vi "Engine-RPC-Host.vi"() -> ()   [LabVIEW 2016]
uses:
  Shared/Typedefs/Engine-RPC-Sync-Controls.ctl
  Shared/Typedefs/Engine-RPC-Sync-Indicators.ctl
  <vilib>/Powertrain Controls/Device Drivers/DCM/Rev0/FPGA/Digital Channel.ctl
  Shared/Typedefs/Engine-RPC-PWM-Controls.ctl
  Shared/Typedefs/Engine-RPC-PWM-Indicators.ctl
  <vilib>/addons/Software Calibration Management/XControls/SubHost.xctl
  Shared/Typedefs/UserParameter-Array.ctl
  Shared/Typedefs/UserParameter.ctl
  Shared/Typedefs/Engine-RPC-Modes.ctl
  Shared/Typedefs/Engine-Channel.ctl
  Shared/DSI-Shared.lvlib
  <vilib>/Powertrain Controls/Device Drivers/DCM/Rev0/FPGA/DCM - FPGA.lvlib
panel:
  in  "Mode":T1
  in  "_Hidden":enum32{"Page 1"}(tab)
  in  "_Refresh":bool
  out "PWM-A_Fault":bool
  out "PWM-B_Fault":bool
  out "Sync-A_Fault":bool
  out "Sync-B_Fault":bool
  out "PWM-A_DisHHChans":sgl[](array[numeric])
  out "PWM-B_DisHHChans":sgl[](array[numeric])
  out "Channels|Names":string[](array[string])
  in  "ENG|RPC|ClearFaults":bool
  out "ENG|RPC|Fault":bool caption="RailP"
  out "ENG|RPC|UserParamNames":string[](array[string])
  in  "ENG|RPC|UserParamValues":sgl[](array[numeric])
  out "ENG|RPC|UserResults":T2=[{"Name"="", "Value"=0.0}, {"Name"="", "Value"=0.0}, {"Name"="", "Value"=0.0}, {"Name"="", "Value"=0.0}, {"Name"="", "Value"=0.0}, {"Name"="", "Value"=0.0}, {"Name"="", "Value"=0.0}, {"Name"="", "Value"=0.0}, {"Name"="", "Value"=0.0}, {"Name"="", "Value"=0.0}, {"Name"="", "Value"=0.0}, {"Name"="", "Value"=0.0}, {"Name"="", "Value"=0.0}, {"Name"="", "Value"=0.0}, {"Name"="", "Value"=0.0}, {"Name"="", "Value"=0.0}, {"Name"="", "Value"=0.0}, {"Name"="", "Value"=0.0}, {"Name"="", "Value"=0.0}, {"Name"="", "Value"=0.0}, {"Name"="", "Value"=0.0}, {"Name"="", "Value"=0.0}, {"Name"="", "Value"=0.0}, {"Name"="", "Value"=0.0}, {"Name"="", "Value"=0.0}, {"Name"="", "Value"=0.0}, {"Name"="", "Value"=0.0}, {"Name"="", "Value"=0.0}, {"Name"="", "Value"=0.0}, {"Name"="", "Value"=0.0}, {"Name"="", "Value"=0.0}, {"Name"="", "Value"=0.0}, {"Name"="", "Value"=0.0}, {"Name"="", "Value"=0.0}, {"Name"="", "Value"=0.0}, {"Name"="", "Value"=0.0}, {"Name"="", "Value"=0.0}, {"Name"="", "Value"=0.0}, {"Name"="", "Value"=0.0}, {"Name"="", "Value"=0.0}, {"Name"="", "Value"=0.0}, {"Name"="", "Value"=0.0}, {"Name"="", "Value"=0.0}, {"Name"="", "Value"=0.0}, {"Name"="", "Value"=0.0}, {"Name"="", "Value"=0.0}, {"Name"="", "Value"=0.0}, {"Name"="", "Value"=0.0}, {"Name"="", "Value"=0.0}, {"Name"="", "Value"=0.0}, {"Name"="", "Value"=0.0}, {"Name"="", "Value"=0.0}, {"Name"="", "Value"=0.0}, {"Name"="", "Value"=0.0}, {"Name"="", "Value"=0.0}, {"Name"="", "Value"=0.0}, {"Name"="", "Value"=0.0}, {"Name"="", "Value"=0.0}, {"Name"="", "Value"=0.0}, {"Name"="", "Value"=0.0}, {"Name"="", "Value"=0.0}, {"Name"="", "Value"=0.0}, {"Name"="", "Value"=0.0}, {"Name"="", "Value"=0.0}, {"Name"="", "Value"=0.0}, {"Name"="", "Value"=0.0}, {"Name"="", "Value"=0.0}, {"Name"="", "Value"=0.0}, {"Name"="", "Value"=0.0}, {"Name"="", "Value"=0.0}, {"Name"="", "Value"=0.0}, {"Name"="", "Value"=0.0}, {"Name"="", "Value"=0.0}, {"Name"="", "Value"=0.0}, {"Name"="", "Value"=0.0}, {"Name"="", "Value"=0.0}, {"Name"="", "Value"=0.0}, {"Name"="", "Value"=0.0}, {"Name"="", "Value"=0.0}, {"Name"="", "Value"=0.0}, {"Name"="", "Value"=0.0}, {"Name"="", "Value"=0.0}, {"Name"="", "Value"=0.0}, {"Name"="", "Value"=0.0}, {"Name"="", "Value"=0.0}, {"Name"="", "Value"=0.0}, {"Name"="", "Value"=0.0}, {"Name"="", "Value"=0.0}, {"Name"="", "Value"=0.0}, {"Name"="", "Value"=0.0}, {"Name"="", "Value"=0.0}, {"Name"="", "Value"=0.0}, {"Name"="", "Value"=0.0}, {"Name"="", "Value"=0.0}, {"Name"="", "Value"=0.0}, {"Name"="", "Value"=0.0}, {"Name"="", "Value"=0.0}, {"Name"="", "Value"=0.0}, {"Name"="", "Value"=0.0}, {"Name"=" ", "Value"=0.0}]
  in  "Rail Pressure Plot":T4(xcontrol)={"Name"="Engine-RPC-Plot-Host (Engine-RPC-Plot-Host)", "Host VI"=path "Engine-RPC-Plot-Host.vi", "Pairing File"=path "Engine-RPC-Plot-Host.par", "Display Name"="Rail Pressure Plot"}
  in  "_RailP Summary Table":i32(listbox) caption="Summary"
  in  "_MainTab":T5(tab)
  in  "PWM-A_Controls":T6
  out "PWM-A_Indicators":T7={"IMV"={"Current_Calc"=0.0, "DutyCyc_PIDOut"=0.7671859, "DutyCyc_MaxCalc"=0.0, "DutyCyc_Des"=0.7671859}, "HPV"={"Current_Calc"=0.0, "DutyCyc_TblOut"=0.7671859, "DutyCyc_MaxCalc"=0.0, "DutyCyc_Des"=0.7671859}} {"HPV"."DutyCyc_Des" format="%#.3g"; "HPV"."DutyCyc_MaxCalc" max=50 format="%#.3g"; "HPV"."DutyCyc_TblOut" format="%#.3g"; "HPV"."Current_Calc" min=0 max=0.2 step=0.001 format="%#.3f"; "IMV"."DutyCyc_Des" format="%#.3g"; "IMV"."DutyCyc_MaxCalc" max=50 format="%#.3g"; "IMV"."DutyCyc_PIDOut" format="%#.3g"; "IMV"."Current_Calc" min=0 max=0.2 step=0.001 format="%#.3f"}
  in  "PWM-A_RailPStp":sgl caption="[bar]"
  out "_PWM-A_SetpointUnit":string
  out "_PWM-A_MaxUnit":string
  in  "PWM-A_MaxRailP":sgl caption="[bar]"
  in  "PWM-A_HPV_E":bool
  in  "PWM-A_IMV_E":bool
  in  "PWM-A_IMVPID_E":bool
  in  "_PWM-A_Tab":enum32{"Analog Inputs", "HH Outputs"}(tab)
  in  "PWM-A_RailPIndex":i32(ring) caption="Select"
  out "PWM-A_RailP":T8 caption="Sensor"
  in  "PWM-A_IMVChannelIndex":i32(ring) items=["Select IMV"=-1, "IMV--HH 1"=0, "IMV--HH 2"=1, "IMV--HH 3"=2, "IMV--HH 4"=3, "IMV--HH 5"=4, "IMV--HH 6"=5, "IMV--HH 7"=6, "IMV--HH 8"=7, "IMV--HH 9"=8, "IMV--HH 10"=9, "IMV--HH 11"=10, "IMV--HH 12"=11]
  in  "PWM-A_HPVChannelIndex":i32(ring) items=["Select HPV"=-1, "HPV--HH 1"=0, "HPV--HH 2"=1, "HPV--HH 3"=2, "HPV--HH 4"=3, "HPV--HH 5"=4, "HPV--HH 6"=5, "HPV--HH 7"=6, "HPV--HH 8"=7, "HPV--HH 9"=8, "HPV--HH 10"=9, "HPV--HH 11"=10, "HPV--HH 12"=11]
  in  "PWM-A PID Settings":T4(xcontrol)
  in  "PWM-B_Controls":T6
  out "PWM-B_Indicators":T7={"IMV"={"Current_Calc"=0.0, "DutyCyc_PIDOut"=0.7671859, "DutyCyc_MaxCalc"=0.0, "DutyCyc_Des"=0.7671859}, "HPV"={"Current_Calc"=0.0, "DutyCyc_TblOut"=0.7671859, "DutyCyc_MaxCalc"=0.0, "DutyCyc_Des"=0.7671859}} {"HPV"."DutyCyc_Des" format="%#.3g"; "HPV"."DutyCyc_MaxCalc" max=50 format="%#.3g"; "HPV"."DutyCyc_TblOut" format="%#.3g"; "HPV"."Current_Calc" min=0 max=0.2 step=0.001 format="%#.3f"; "IMV"."DutyCyc_Des" format="%#.3g"; "IMV"."DutyCyc_MaxCalc" max=50 format="%#.3g"; "IMV"."DutyCyc_PIDOut" format="%#.3g"; "IMV"."Current_Calc" min=0 max=0.2 step=0.001 format="%#.3f"}
  in  "PWM-B_RailPStp":sgl caption="[bar]"
  out "_PWM-B_SetpointUnit":string
  out "_PWM-B_MaxUnit":string
  in  "PWM-B_MaxRailP":sgl caption="[bar]"
  in  "PWM-B_HPV_E":bool
  in  "PWM-B_IMV_E":bool
  in  "PWM-B_IMVPID_E":bool
  in  "_PWM-B_Tab":enum32{"Analog Inputs", "HH Outputs"}(tab)
  in  "PWM-B_RailPIndex":i32(ring) caption="Select"
  out "PWM-B_RailP":T8 caption="Sensor"
  in  "PWM-B_IMVChannelIndex":i32(ring) items=["Select IMV"=-1, "IMV--HH 1"=0, "IMV--HH 2"=1, "IMV--HH 3"=2, "IMV--HH 4"=3, "IMV--HH 5"=4, "IMV--HH 6"=5, "IMV--HH 7"=6, "IMV--HH 8"=7, "IMV--HH 9"=8, "IMV--HH 10"=9, "IMV--HH 11"=10, "IMV--HH 12"=11]
  in  "PWM-B_HPVChannelIndex":i32(ring) items=["Select HPV"=-1, "HPV--HH 1"=0, "HPV--HH 2"=1, "HPV--HH 3"=2, "HPV--HH 4"=3, "HPV--HH 5"=4, "HPV--HH 6"=5, "HPV--HH 7"=6, "HPV--HH 8"=7, "HPV--HH 9"=8, "HPV--HH 10"=9, "HPV--HH 11"=10, "HPV--HH 12"=11]
  in  "PWM-B PID Settings":T4(xcontrol)
  in  "Sync-A_Controls":T9 {"Timing"."MinOffTime" format="%#.2f"; "Timing"."DurAngle_Max" format="%#.2f"; "Timing"."WindowEnd" format="%#.2f"; "Timing"."WindowStart" format="%#.2f"; "Duration"."Dur_Man" format="%#.2f"; "Duration"."Dur_Min" format="%#.2f"; "Duration"."Dur_Max" format="%#.2f"}
  in  "Sync-A_Timing_EPT":sgl caption="[DBTDC]"
  in  "Sync-A_TimingMode":bool
  in  "Sync-A_DurPID_E":bool
  in  "Sync-A_Ctrl_E":bool
  in  "Sync-A_MaxRailP":sgl caption="[bar]"
  out "_Sync-A_MaxUnit":string
  out "_Sync-A_SetpointUnit":string
  in  "Sync-A_RailPStp":sgl caption="[bar]"
  out "Sync-A_Indicators":T10
  in  "Sync-A_Timing_TMP":sgl caption="[%]"
  in  "_Sync-A_Tab":enum32{"Analog Inputs", "Digital Inputs"}(tab)
  in  "Sync-A_RailPIndex":i32(ring) caption="Select"
  out "Sync-A_RailP":T8 caption="Sensor"
  in  "Sync-A_CamLobes":u8
  in  "Sync-A_CamDefaultPsn":sgl caption="[DBTDC]"
  in  "Sync-A_DigitalInput":T11 caption="Select"
  in  "Sync-A PID Settings":T4(xcontrol)
  in  "Sync-B_Controls":T9 {"Timing"."MinOffTime" format="%#.2f"; "Timing"."DurAngle_Max" format="%#.2f"; "Timing"."WindowEnd" format="%#.2f"; "Timing"."WindowStart" format="%#.2f"; "Duration"."Dur_Man" format="%#.2f"; "Duration"."Dur_Min" format="%#.2f"; "Duration"."Dur_Max" format="%#.2f"}
  in  "Sync-B_Timing_EPT":sgl caption="[DBTDC]"
  in  "Sync-B_TimingMode":bool
  in  "Sync-B_DurPID_E":bool
  in  "Sync-B_Ctrl_E":bool
  in  "Sync-B_MaxRailP":sgl caption="[bar]"
  out "_Sync-B_MaxUnit":string
  out "_Sync-B_SetpointUnit":string
  in  "Sync-B_RailPStp":sgl caption="[bar]"
  out "Sync-B_Indicators":T10
  in  "Sync-B_Timing_TMP":sgl caption="[%]"
  in  "_Sync-B_Tab":enum32{"Analog Inputs", "Digital Inputs"}(tab)
  in  "Sync-B_RailPIndex":i32(ring) caption="Select"
  out "Sync-B_RailP":T8 caption="Sensor"
  in  "Sync-B_CamLobes":u8
  in  "Sync-B_CamDefaultPsn":sgl caption="[DBTDC]"
  in  "Sync-B_DigitalInput":T11 caption="Select"
  in  "Sync-B PID Settings":T4(xcontrol)
  in  "_User Param":string[][](table) caption="User Parameters"
  out "_User Results":string[][](table) caption="User Results"
  in  "UserVI_Reload":bool
  in  "UserVI_Filename":string caption="User Plugin File Path (.lvclass relative to default data directory)"
  out "PluginError":bool caption="User VI Error"
  # "Rail Pressure Control"
  # "Control Mode"
  # "PWM Common Rail Pump - Bank A"
  # "RailPStp"
  # "MaxRailP"
  # "Input"
  # "PWM Common Rail Pump - Bank B"
  # "RailPStp"
  # "MaxRailP"
  # "Input"
  # "Synchronous Common Rail Pump - Bank A"
  # "RailPStp"
  # "MaxRailP"
  # "Input"
  # "Synchronous Common Rail Pump - Bank B"
  # "RailPStp"
  # "MaxRailP"
  # "Input"
  # "User VI"
  # "User Plugin File Path (.lvclass relative to default data directory)"
types:
  T1 = typedef "DSI-Shared.lvlib/Engine-RPC-Modes.ctl" = enum8{"Disabled", "DSI - PWM Pumps", "DSI - Sync Pumps", "User Plugin"}
  T2 = typedef "DSI-Shared.lvlib/UserParameter-Array.ctl" = T3[]
  T3 = typedef "DSI-Shared.lvlib/UserParameter.ctl" = cluster{"Name":string, "Value":dbl}
  T4 = cluster{"Name":string, "Host VI":path, "Pairing File":path, "Display Name":string}
  T5 = enum32{"PWM Pump A", "PWM Pump B", "Sync Pump A", "Sync Pump B", "User Plugin"}
  T6 = typedef "DSI-Shared.lvlib/Engine-RPC-PWM-Controls.ctl" = cluster{"IMV":cluster{"PWMFreq":sgl, "NomResistance":sgl, "DutyCyc_Max":sgl, "Min Duty Cycle":sgl, "DutyCycle_ManE":bool, "DutyCycle_Man":sgl}, "HPV":cluster{"PWMFreq":sgl, "NomResistance":sgl, "DutyCyc_Max":sgl, "Min Duty Cycle":sgl, "DutyCycle_ManE":bool, "DutyCycle_Man":sgl}}
  T7 = typedef "DSI-Shared.lvlib/Engine-RPC-PWM-Indicators.ctl" = cluster{"IMV":cluster{"Current_Calc":sgl, "DutyCyc_PIDOut":sgl, "DutyCyc_MaxCalc":sgl, "DutyCyc_Des":sgl}, "HPV":cluster{"Current_Calc":sgl, "DutyCyc_TblOut":sgl, "DutyCyc_MaxCalc":sgl, "DutyCyc_Des":sgl}}
  T8 = cluster{"Name":string, "Unit":string, "Value":sgl}
  T9 = typedef "DSI-Shared.lvlib/Engine-RPC-Sync-Controls.ctl" = cluster{"Duration":cluster{"Dur_Max":sgl, "Dur_Min":sgl, "Dur_ManE":bool, "Dur_Man":sgl}, "Timing":cluster{"WindowStart":sgl, "WindowEnd":sgl, "EndAngle?":bool, "DurAngle_Max":sgl, "MinOffTime":sgl}}
  T10 = typedef "DSI-Shared.lvlib/Engine-RPC-Sync-Indicators.ctl" = cluster{"Duration":cluster{"Duration_Output":sgl, "PID_Output":sgl}, "EPT Mode":cluster{"Sync-A_Timing":sgl, "Sync-A_CamAdv":sgl}, "TMP Mode":cluster{"Sync-A_Delay":sgl, "Sync-A_Period":sgl}}
  T11 = typedef "DCM - FPGA.lvlib/Digital Channel.ctl" = enum8{"Unused", "Diff IO 1", "Diff IO 2", "Diff IO 3", "Diff IO 4", "Diff IO 5", "Diff IO 6", "Diff IO 7", "Diff IO 8", "Aux 1", "Aux 2", "Aux 3", "Aux 4", "Aux 5", "Aux 6", "Aux 7", "Aux 8", "User OS"}
  T12 = enum32{"Invalid", "Standard", "Closed", "Hidden", "Minimized", "Maximized"}
  T13 = typedef "DSI-Shared.lvlib/Engine-Channel.ctl" = cluster{"Name":string, "Unit":string, "Value":sgl}
  T14 = cluster{"Sensor":T13, "Setpoint":sgl, "Timing Mode":bool, "Timing_EPT":sgl, "Timing_TMP":sgl, "Sync-A_Indicators":T10, "Fault":bool, "Enable":bool}
  T15 = cluster{"Sensor":T13, "Setpoint":sgl, "PWM-A_Indicators":T7, "PWM-A_IMVChannelIndex":i32, "PWM-A_HPVChannelIndex":i32, "Fault":bool, "Enable":bool}
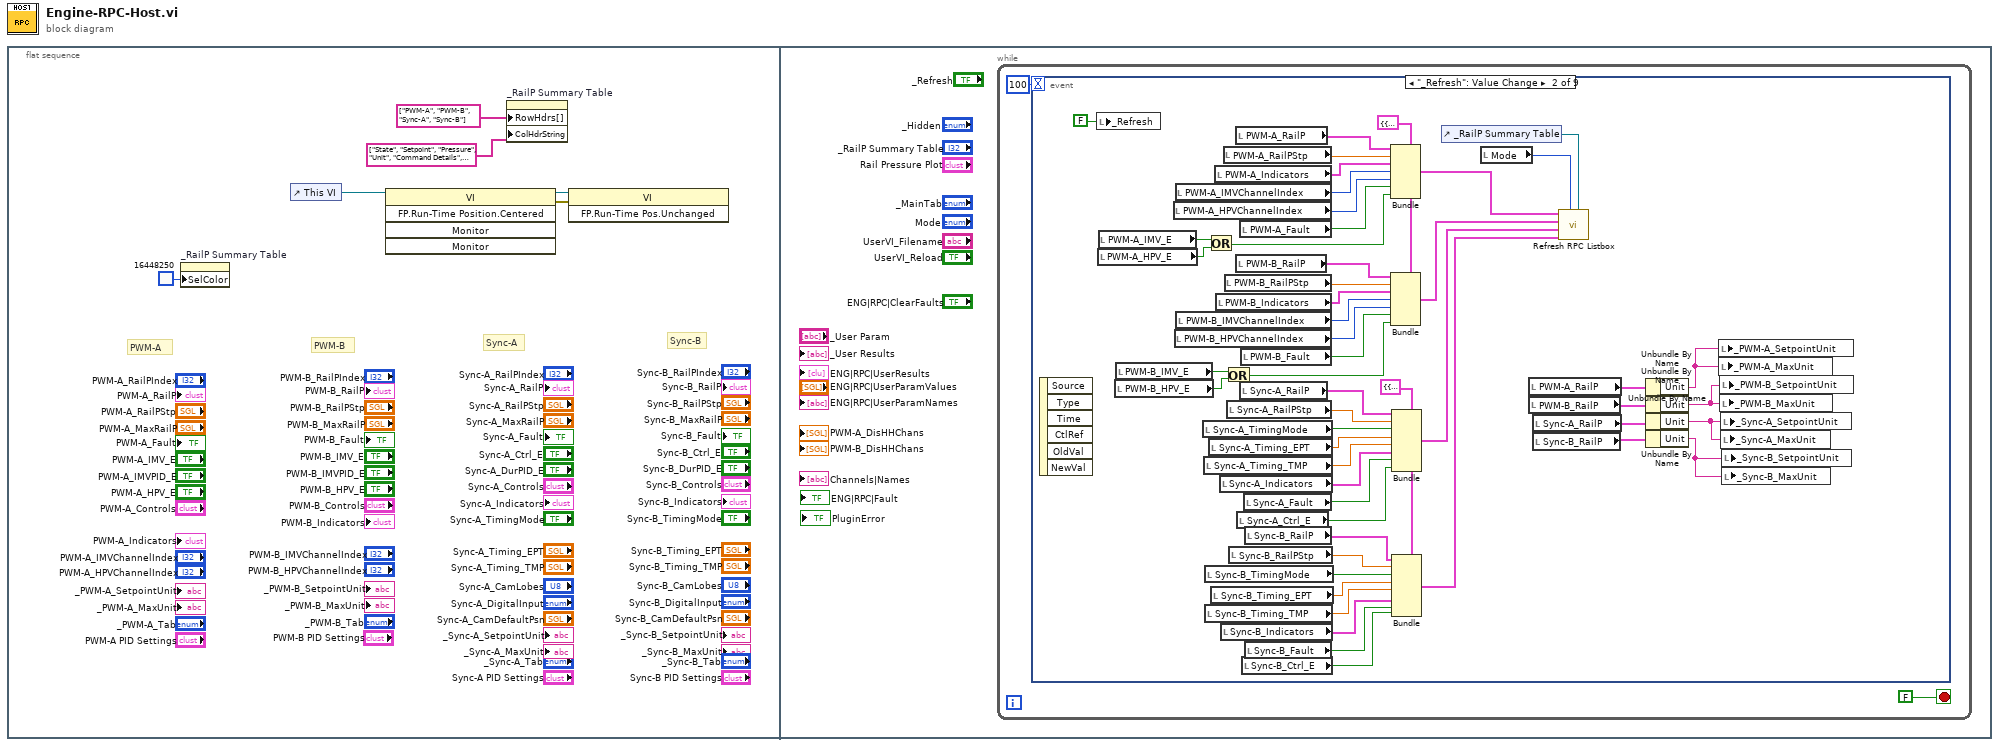
[diagram p0: block diagram]
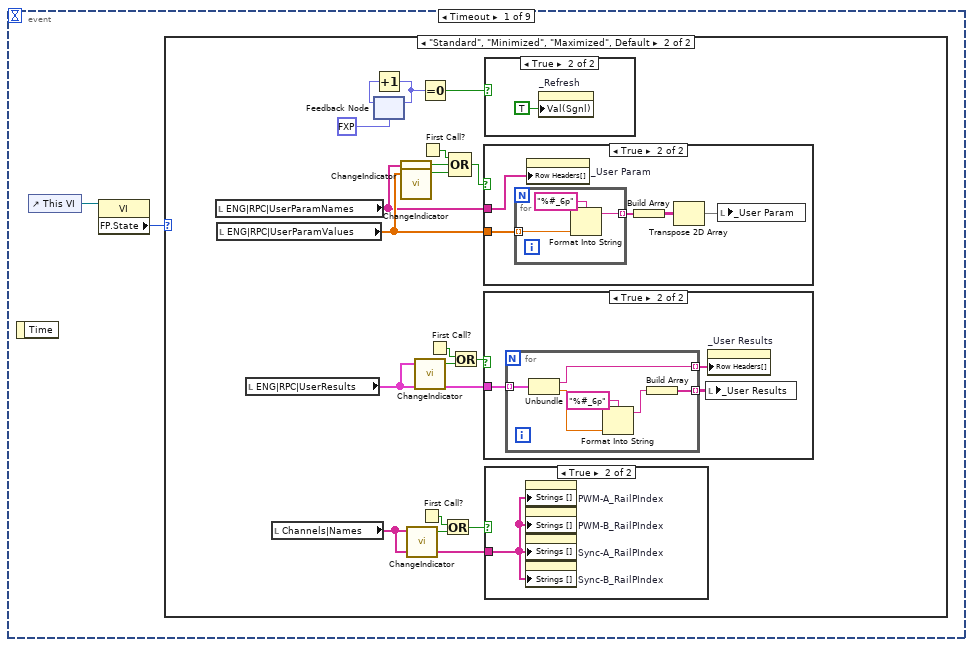
[diagram p2: hidden frame]
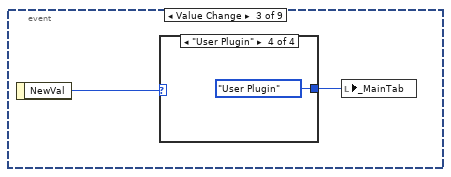
[diagram p8: hidden frame]
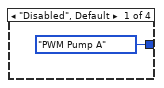
[diagram p9: hidden frame]
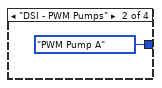
[diagram p10: hidden frame]
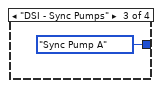
[diagram p11: hidden frame]
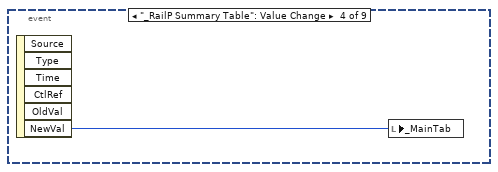
[diagram p12: hidden frame]
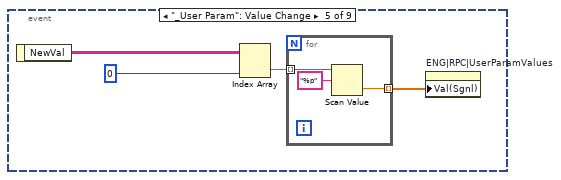
[diagram p13: hidden frame]
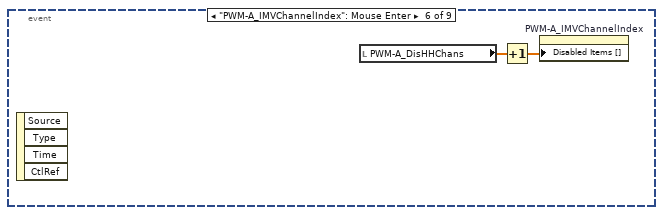
[diagram p14: hidden frame]
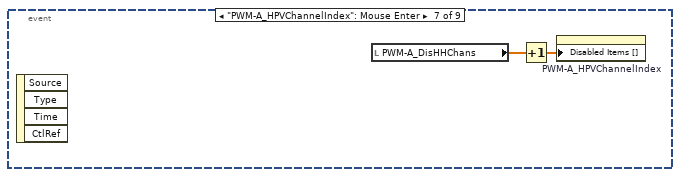
[diagram p15: hidden frame]
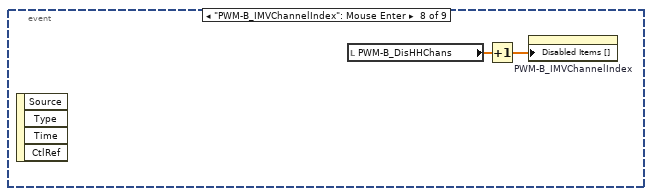
[diagram p16: hidden frame]
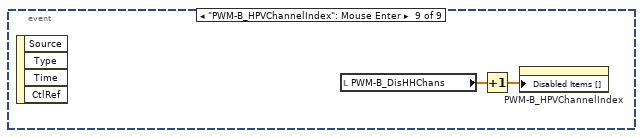
[diagram p17: hidden frame]
diagram:
  n1 = flat-sequence {
    frame #0 {
      # "Sync-B"
      # "Sync-A"
      # "PWM-B"
      # "PWM-A"
      n2 = property on="_RailP Summary Table" class="MCListbox (strict)"("SelColor"=u32 16448250 ("Selection Color")) -> ()  [unwired: 2 in, 2 out]
      n3 = control-ref of="This VI"() -> (w4:refnum<vi>)
      n4 = invoke class="VI" method="FP.Run-Time Position.Centered"(reference=w4) -> (reference out=w5:refnum<vi>, error out=w6:errorcluster)  [unwired: 4 in, 3 out]
      n5 = property on="_RailP Summary Table" class="MCListbox (strict)"("RowHdrs[]"=string[] ["PWM-A", "PWM-B", "Sync-A", "Sync-B"] ("Row Header Strings[]"), "ColHdrString"=string[] ["State", "Setpoint", "Pressure", "Unit", "Command Details", "Fault"] ("Column Header Strings[]")) -> ()  [unwired: 2 in, 2 out]
      n6 = invoke class="VI" method="FP.Run-Time Pos.Unchanged"(reference=w5, error in=w6) -> ()  [unwired: 1 in, 3 out]
    }
    frame #1 {
      n7 = while {
        stop <- FALSE stop-if-true
        n8 = event shown="[1] \"_Refresh\": Value Change" {
          selector: _ -> [_ _ _ _ _ _ _ _ _]
          dyn-events: _ -> [_ _ _ _ _ _ _ _ _]
          timeout: 100 ("milliseconds to wait") -> [_ _ _ _ _ _ _ _ _]
          event Timeout {
            n9 = event-data() -> ()  [unwired: 1 in, 1 out]
            n10 = control-ref of="This VI"() -> (w10:refnum<vi>)
            n11 = property class="VI"(reference=w10) -> ("FP.State"=w9:T12)  [unwired: 1 in, 2 out]
            n12 = case shown="\"Standard\", \"Minimized\", \"Maximized\", Default" w9 {
              frame "Invalid", "Closed", "Hidden" {
              }
              frame "Standard", "Minimized", "Maximized", Default {
                n13 = local read "ENG|RPC|UserParamNames"() -> (w26:string[])
                n14 = local read "ENG|RPC|UserParamValues"() -> (w27:sgl[])
                n15 = local read "ENG|RPC|UserResults"() -> (w19:T2)
                n16 = local read "Channels|Names"() -> (w15:string[])
                n17 = feedback #1(fxp<+,1,4> 0.0) -> (w13:fxp<+,1,4>)
                n18 = Increment(x=w13) -> (x+1=w12:fxp<+,1,4>)
                n19 = feedback-in #1(w12) -> ()
                n20 = call "ChangeIndicator.vi"("Input"=w26) -> ("Change"=w25:bool)  [unwired: 9 in]
                n21 = call "ChangeIndicator.vi"("Input"=w27) -> ("Change"=w23:bool)  [unwired: 9 in]
                n22 = call "ChangeIndicator.vi"("Input"=w15) -> ("Change"=w18:bool)  [unwired: 9 in]
                n23 = call "ChangeIndicator.vi"("Input"=w19) -> ("Change"=w20:bool)  [unwired: 9 in]
                n24 = First Call?() -> (First Call?: T/F=w17:bool)
                n25 = First Call?() -> (First Call?: T/F=w28:bool)
                n26 = Equal To 0?(x=w12) -> (x = 0?=w11:bool)
                n27 = First Call?() -> (First Call?: T/F=w22:bool)
                n28 = Or(x=w17, y=w18) -> (x .or. y?=w16:bool)
                n29 = Compound Arithmetic op=OR(w28, w25, w23) -> (w24:bool)
                n30 = Or(x=w22, y=w20) -> (x .or. y?=w21:bool)
                n31 = case shown="True" w24 {
                  tunnel: w26 -> [_ w42]
                  tunnel: w27 -> [_ w41]
                  frame False {
                  }
                  frame True {
                    n32 = for {
                      tunnel: w41 -> [w47] mode=indexing
                      tunnel: [w46] -> w40 mode=indexing
                      n33 = Format Into String(format string="%#_6p", w47) -> (resulting string=w46:string)  [unwired: 2 in, 1 out]
                    }
                    n34 = property on="_User Param" class="Tbl (strict)"("Row Headers[]"=w42) -> ()  [unwired: 2 in, 2 out]
                    n35 = Build Array(w40) -> (w43:string[][])
                    n36 = Transpose 2D Array(2D array=w43) -> (transposed array=w44:string[][])
                    n37 = local write "_User Param"(w44) -> ()
                  }
                }
                n38 = case shown="True" w21 {
                  tunnel: w19 -> [_ w32]
                  frame False {
                  }
                  frame True {
                    n39 = for {
                      tunnel: w32 -> [w39] mode=indexing
                      tunnel: [w38] -> w33 mode=indexing
                      tunnel: [w37] -> w31 mode=indexing
                      n40 = Unbundle(w39) -> ("Name"=w37:string, "Value"=w35:dbl)
                      n41 = Format Into String(format string="%#_6p", w35) -> (resulting string=w34:string)  [unwired: 2 in, 1 out]
                      n42 = Build Array(w34) -> (w38:string[])
                    }
                    n43 = local write "_User Results"(w33) -> ()
                    n44 = property on="_User Results" class="Tbl (strict)"("Row Headers[]"=w31) -> ()  [unwired: 2 in, 2 out]
                  }
                }
                n45 = case shown="True" w11 {
                  frame False {
                  }
                  frame True {
                    n46 = property on="_Refresh" class="Bool (strict)"("Val(Sgnl)"=TRUE ("Value (Signaling)")) -> ()  [unwired: 2 in, 2 out]
                  }
                }
                n47 = case shown="True" w16 {
                  tunnel: w15 -> [_ w30]
                  frame False {
                  }
                  frame True {
                    n48 = property on="PWM-A_RailPIndex" class="Ring (strict)"("Strings []"=w30) -> ()  [unwired: 2 in, 2 out]
                    n49 = property on="PWM-B_RailPIndex" class="Ring (strict)"("Strings []"=w30) -> ()  [unwired: 2 in, 2 out]
                    n50 = property on="Sync-A_RailPIndex" class="Ring (strict)"("Strings []"=w30) -> ()  [unwired: 2 in, 2 out]
                    n51 = property on="Sync-B_RailPIndex" class="Ring (strict)"("Strings []"=w30) -> ()  [unwired: 2 in, 2 out]
                  }
                }
              }
            }
          }
          event "_Refresh": Value Change {
            w66 = T14 {"Sensor"={"Name"="", "Unit"="", "Value"=0.0}, "Setpoint"=0.0, "Timing Mode"=FALSE, "Timing_EPT"=0.0, "Timing_TMP"=0.0, "Sync-A_Indicators"={"Duration"={"Duration_Output"=0.0, "PID_Output"=0.0}, "EPT Mode"={"Sync-A_Timing"=0.0, "Sync-A_CamAdv"=0.0}, "TMP Mode"={"Sync-A_Delay"=0.0, "Sync-A_Period"=0.0}}, "Fault"=FALSE, "Enable"=FALSE} ("Sync-B")
            w68 = T15 {"Sensor"={"Name"="", "Unit"="", "Value"=0.0}, "Setpoint"=0.0, "PWM-A_Indicators"={"IMV"={"Current_Calc"=0.0, "DutyCyc_PIDOut"=0.7671859, "DutyCyc_MaxCalc"=0.0, "DutyCyc_Des"=0.7671859}, "HPV"={"Current_Calc"=0.0, "DutyCyc_TblOut"=0.7671859, "DutyCyc_MaxCalc"=0.0, "DutyCyc_Des"=0.7671859}}, "PWM-A_IMVChannelIndex"=0, "PWM-A_HPVChannelIndex"=0, "Fault"=FALSE, "Enable"=FALSE} ("PWM-A")
            n52 = event-data() -> ()  [unwired: 1 in, 6 out]
            n53 = local write "_Refresh"(FALSE ("_Refresh")) -> ()
            n54 = local read "PWM-A_HPV_E"() -> (w51:bool)
            n55 = local read "PWM-A_IMV_E"() -> (w52:bool)
            n56 = local read "PWM-B_HPV_E"() -> (w50:bool)
            n57 = local read "PWM-B_IMV_E"() -> (w49:bool)
            n58 = local read "PWM-A_HPVChannelIndex"() -> (w93:i32)
            n59 = local read "PWM-B_HPVChannelIndex"() -> (w88:i32)
            n60 = local read "PWM-A_IMVChannelIndex"() -> (w92:i32)
            n61 = local read "PWM-B_IMVChannelIndex"() -> (w89:i32)
            n62 = local read "Sync-A_TimingMode"() -> (w80:bool)
            n63 = local read "Sync-A_Timing_TMP"() -> (w78:sgl)
            n64 = local read "Sync-B_TimingMode"() -> (w73:bool)
            n65 = local read "Sync-B_Timing_TMP"() -> (w71:sgl)
            n66 = Or(x=w52, y=w51) -> (x .or. y?=w53:bool)
            n67 = local read "Sync-A_Timing_EPT"() -> (w79:sgl)
            n68 = local read "Sync-B_Timing_EPT"() -> (w72:sgl)
            n69 = local read "PWM-A_Indicators"() -> (w94:T7)
            n70 = local read "PWM-B_Indicators"() -> (w87:T7)
            n71 = local read "Sync-A_Indicators"() -> (w77:T10)
            n72 = local read "Sync-B_Indicators"() -> (w70:T10)
            n73 = local read "PWM-A_RailPStp"() -> (w95:sgl)
            n74 = local read "PWM-B_RailPStp"() -> (w86:sgl)
            n75 = Or(x=w49, y=w50) -> (x .or. y?=w48:bool)
            n76 = local read "Sync-A_RailPStp"() -> (w81:sgl)
            n77 = local read "Sync-B_RailPStp"() -> (w74:sgl)
            n78 = local read "PWM-A_RailP"() -> (w96:T8)
            n79 = local read "PWM-B_RailP"() -> (w85:T8)
            n80 = local read "Sync-A_Ctrl_E"() -> (w63:bool)
            n81 = local read "PWM-A_Fault"() -> (w91:bool)
            n82 = local read "Sync-A_RailP"() -> (w82:T8)
            n83 = local read "PWM-B_Fault"() -> (w90:bool)
            n84 = local read "Sync-B_Ctrl_E"() -> (w64:bool)
            n85 = local read "Sync-A_Fault"() -> (w76:bool)
            n86 = local read "Sync-B_RailP"() -> (w75:T8)
            n87 = local read "Sync-B_Fault"() -> (w69:bool)
            n88 = Bundle(cluster=w68, "Sensor"=w96, "Setpoint"=w95, "PWM-A_Indicators"=w94, "PWM-A_IMVChannelIndex"=w92, "PWM-A_HPVChannelIndex"=w93, "Fault"=w91, "Enable"=w53) -> (w67:T15)
            n89 = Bundle(cluster=w68, "Sensor"=w85, "Setpoint"=w86, "PWM-A_Indicators"=w87, "PWM-A_IMVChannelIndex"=w89, "PWM-A_HPVChannelIndex"=w88, "Fault"=w90, "Enable"=w48) -> (w84:T15)
            n90 = Bundle(cluster=w66, "Sensor"=w82, "Setpoint"=w81, "Timing Mode"=w80, "Timing_EPT"=w79, "Timing_TMP"=w78, "Sync-A_Indicators"=w77, "Fault"=w76, "Enable"=w63) -> (w83:T14)
            n91 = Bundle(cluster=w66, "Sensor"=w75, "Setpoint"=w74, "Timing Mode"=w73, "Timing_EPT"=w72, "Timing_TMP"=w71, "Sync-A_Indicators"=w70, "Fault"=w69, "Enable"=w64) -> (w65:T14)
            n92 = control-ref of="_RailP Summary Table"() -> (w97:refnum<vi>)
            n93 = local read "Mode"() -> (w62:T1)
            n94 = local read "PWM-A_RailP"() -> (w61:T8)
            n95 = local read "PWM-B_RailP"() -> (w60:T8)
            n96 = local read "Sync-A_RailP"() -> (w59:T8)
            n97 = local read "Sync-B_RailP"() -> (w58:T8)
            n98 = call "Refresh RPC Listbox.vi"("_RailP Summary Table"=w97, "Mode"=w62, "Sync-B"=w65, "Sync-A"=w83, "PWM-B"=w84, "PWM-A"=w67) -> ()  [unwired: 6 in]
            n99 = Unbundle By Name(w61) -> ("Unit"=w57:string)
            n100 = Unbundle By Name(w60) -> ("Unit"=w56:string)
            n101 = Unbundle By Name(w59) -> ("Unit"=w55:string)
            n102 = Unbundle By Name(w58) -> ("Unit"=w54:string)
            n103 = local write "_PWM-A_SetpointUnit"(w57) -> ()
            n104 = local write "_PWM-A_MaxUnit"(w57) -> ()
            n105 = local write "_PWM-B_SetpointUnit"(w56) -> ()
            n106 = local write "_PWM-B_MaxUnit"(w56) -> ()
            n107 = local write "_Sync-A_SetpointUnit"(w55) -> ()
            n108 = local write "_Sync-A_MaxUnit"(w55) -> ()
            n109 = local write "_Sync-B_SetpointUnit"(w54) -> ()
            n110 = local write "_Sync-B_MaxUnit"(w54) -> ()
          }
          event Value Change {
            n111 = event-data() -> ("NewVal"=w100:T1)  [unwired: 1 in]
            n112 = case shown="\"User Plugin\"" w100 {
              tunnel: [T5."PWM Pump A" ("_MainTab") T5."PWM Pump A" ("_MainTab") T5."Sync Pump A" ("_MainTab") T5."User Plugin" ("_MainTab")] -> w99
              frame "Disabled", Default {
              }
              frame "DSI - PWM Pumps" {
              }
              frame "DSI - Sync Pumps" {
              }
              frame "User Plugin" {
              }
            }
            n113 = local write "_MainTab"(w99) -> ()
          }
          event "_RailP Summary Table": Value Change {
            n114 = event-data() -> ("NewVal"=w105:i32)  [unwired: 1 in, 5 out]
            n115 = local write "_MainTab"(w105) -> ()
          }
          event "_User Param": Value Change {
            n116 = event-data() -> ("NewVal"=w109:string[][])  [unwired: 1 in]
            n117 = Index Array(array=w109, index (col)=0 ("disabled index (col)")) -> (element=w107:string[])  [unwired: 1 in]
            n118 = for {
              tunnel: [w112] -> w106 mode=indexing
              tunnel: w107 -> [w111] mode=indexing
              n119 = Scan Value(string=w111, format string="%p") -> (value=w112:dbl)  [unwired: 1 in, 1 out]
            }
            n120 = property on="ENG|RPC|UserParamValues" class="Arr (strict)"("Val(Sgnl)"=w106) -> ()  [unwired: 2 in, 2 out]
          }
          event "PWM-A_IMVChannelIndex": Mouse Enter {
            n121 = event-data() -> ()  [unwired: 1 in, 4 out]
            n122 = local read "PWM-A_DisHHChans"() -> (w114:sgl[])
            n123 = Increment(x=w114) -> (x+1=w113:sgl[])
            n124 = property on="PWM-A_IMVChannelIndex" class="Ring (strict)"("Disabled Items []"=w113) -> ()  [unwired: 2 in, 2 out]
          }
          event "PWM-A_HPVChannelIndex": Mouse Enter {
            n125 = event-data() -> ()  [unwired: 1 in, 4 out]
            n126 = local read "PWM-A_DisHHChans"() -> (w116:sgl[])
            n127 = Increment(x=w116) -> (x+1=w115:sgl[])
            n128 = property on="PWM-A_HPVChannelIndex" class="Ring (strict)"("Disabled Items []"=w115) -> ()  [unwired: 2 in, 2 out]
          }
          event "PWM-B_IMVChannelIndex": Mouse Enter {
            n129 = event-data() -> ()  [unwired: 1 in, 4 out]
            n130 = local read "PWM-B_DisHHChans"() -> (w118:sgl[])
            n131 = Increment(x=w118) -> (x+1=w117:sgl[])
            n132 = property on="PWM-B_IMVChannelIndex" class="Ring (strict)"("Disabled Items []"=w117) -> ()  [unwired: 2 in, 2 out]
          }
          event "PWM-B_HPVChannelIndex": Mouse Enter {
            n133 = event-data() -> ()  [unwired: 1 in, 4 out]
            n134 = local read "PWM-B_DisHHChans"() -> (w120:sgl[])
            n135 = Increment(x=w120) -> (x+1=w119:sgl[])
            n136 = property on="PWM-B_HPVChannelIndex" class="Ring (strict)"("Disabled Items []"=w119) -> ()  [unwired: 2 in, 2 out]
          }
        }
      }
    }
  }
